vi "Loop Time Const.vi"() -> (1 "loop time ms":i64=200)   [LabVIEW 2019]
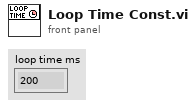
[diagram p1: front panel]
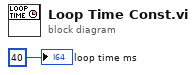
[diagram p0: block diagram]
diagram:
  "loop time ms" <- i64 40
